vi "Drawer.vi"() -> ()   [LabVIEW 2014]
uses:
  <vilib>/Utility/file.llb/Read From Spreadsheet File (string).vi
  <vilib>/Utility/file.llb/Read From Spreadsheet File (I64).vi
  <vilib>/Utility/file.llb/Read From Spreadsheet File (DBL).vi
  <vilib>/Utility/file.llb/Write To Spreadsheet File (DBL).vi
  <vilib>/gmath/NI_Gmath.lvlib
panel:
  out "HF/LF slope":cluster{dbl[], dbl[]}[](graph)
  out "HF/LF flat":cluster{dbl[], dbl[]}[](graph)
  out "HF/LF_ERP 2":i32[][](graph)
  out "HF/LF_ERP":dbl[][](graph)
  out "HF_ERP":dbl[][](graph)
  out "LF_ERP":dbl[][](graph)
  out "VLF_ERP":dbl[][](graph)
  out "피험자_이름":string
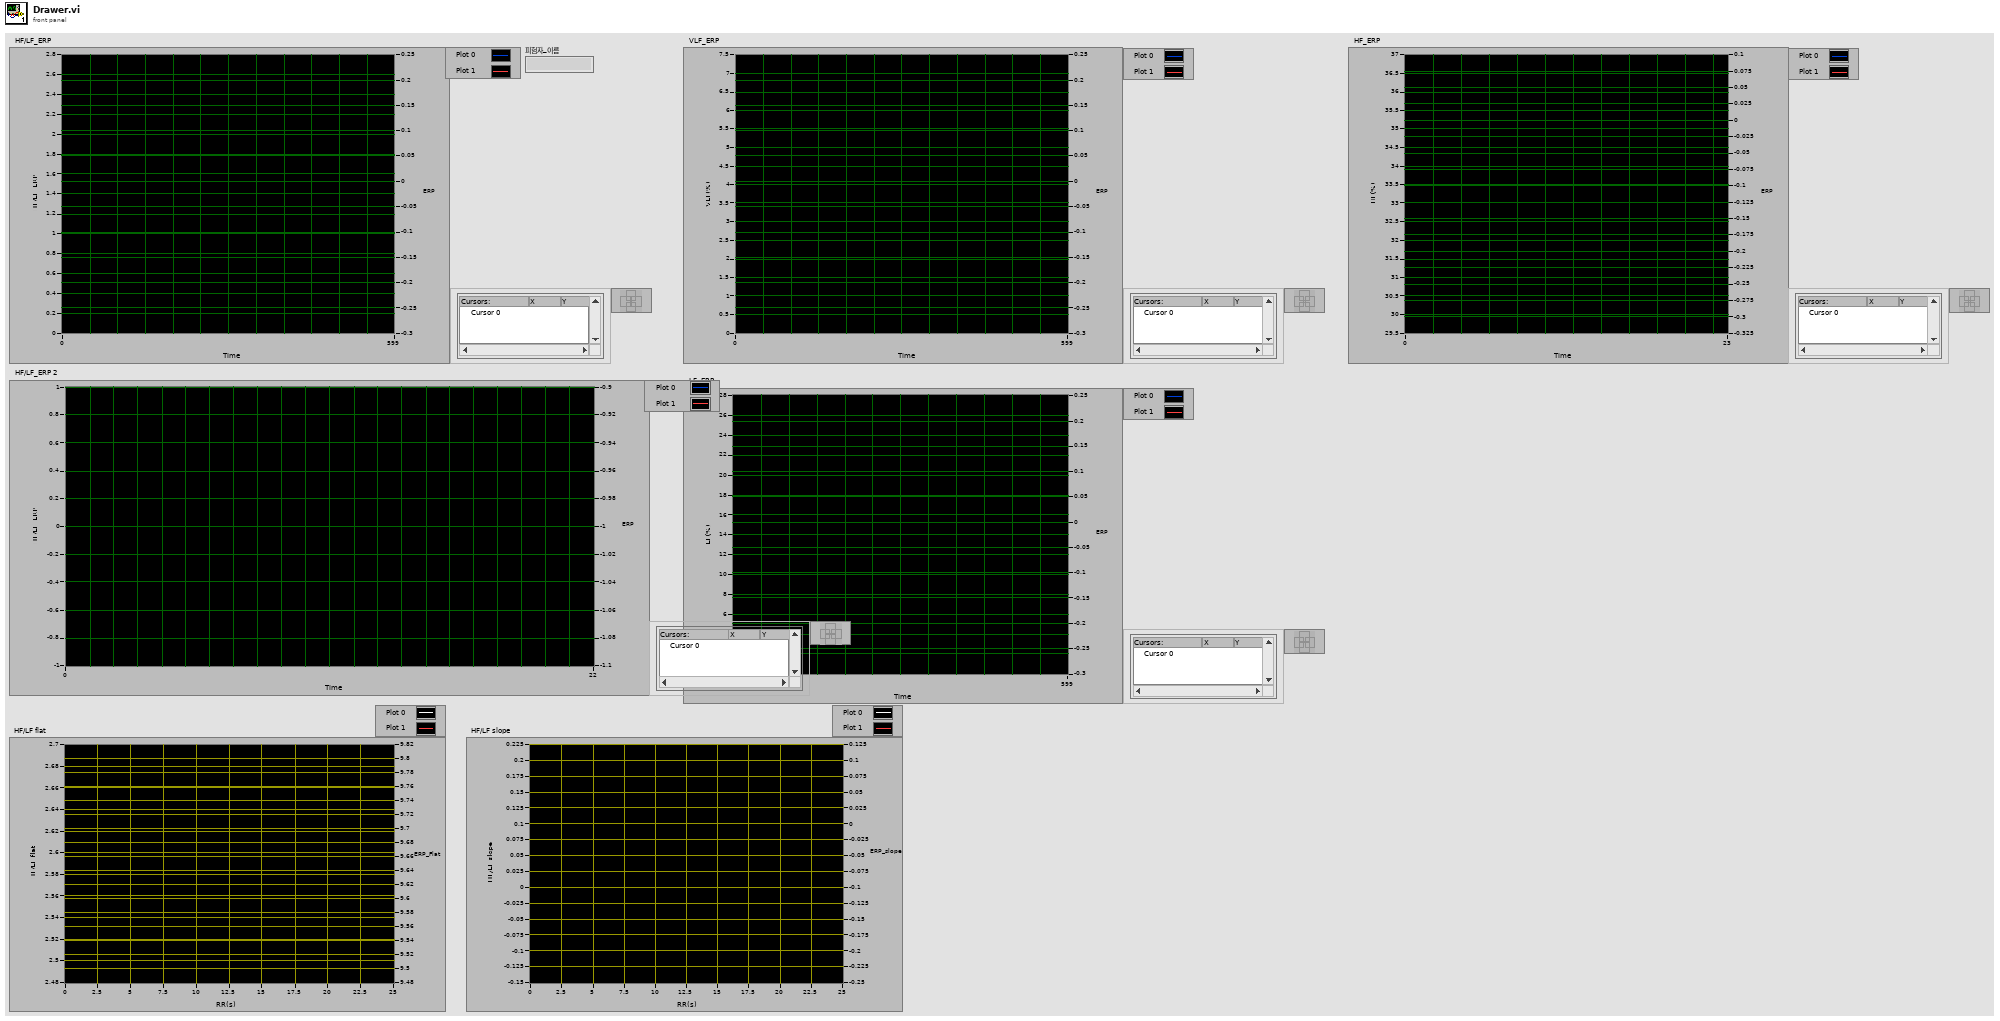
[diagram p1: front panel]
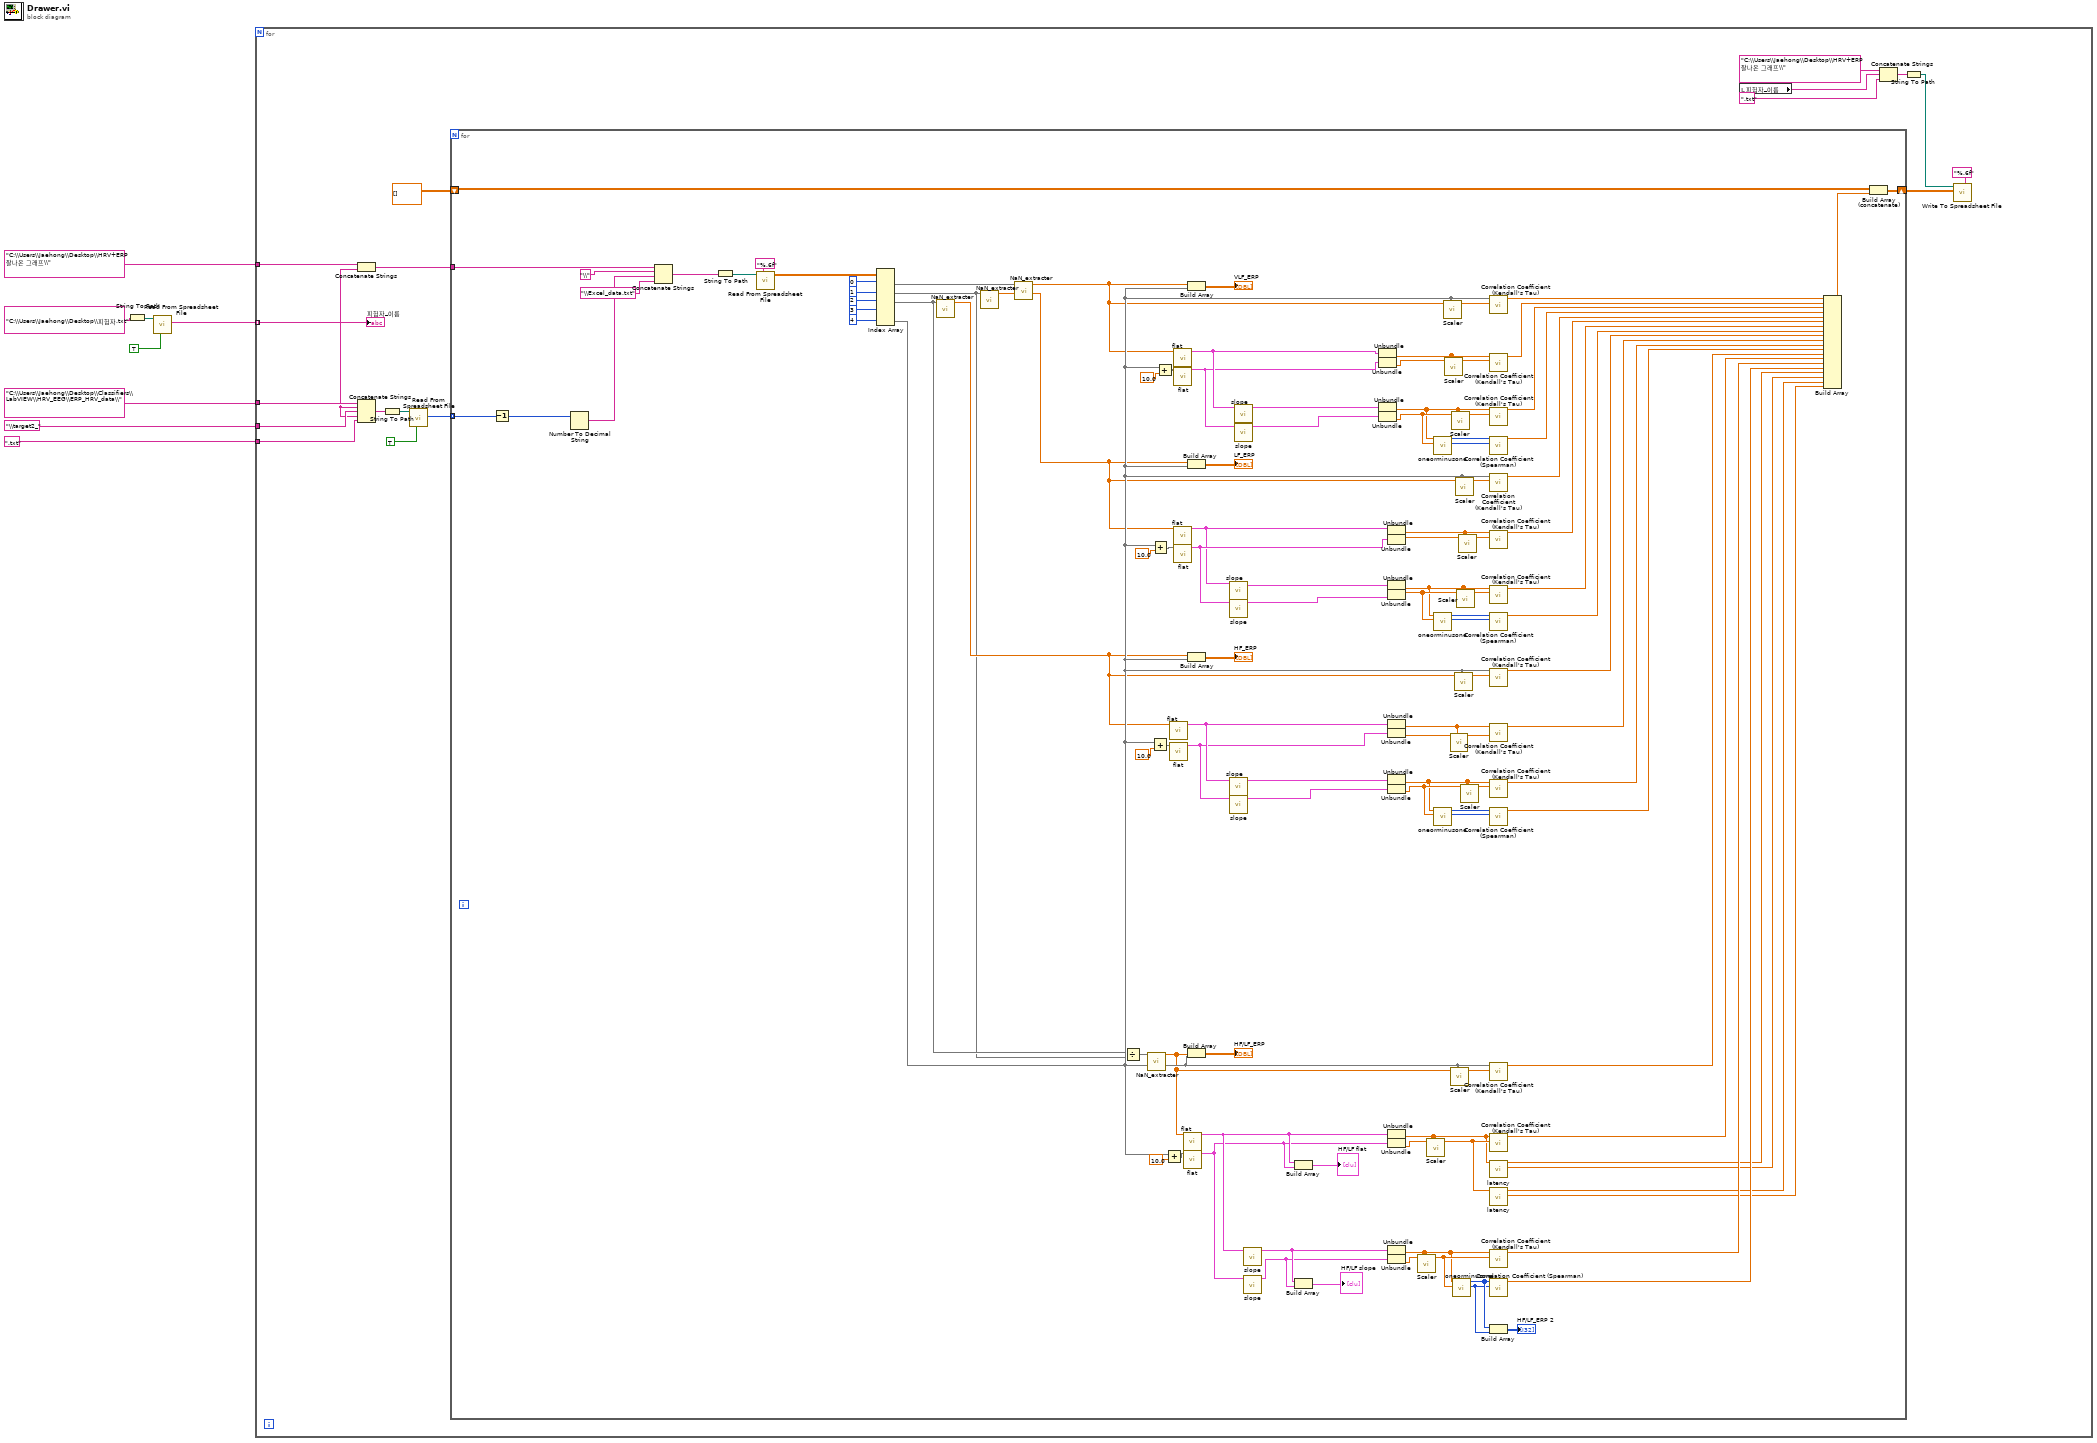
[diagram p0: block diagram]
diagram:
  n1 = String To Path(string="C:\\Users\\Jaehong\\Desktop\\피험자.txt") -> (path=w1:path)
  n2 = call-poly <vilib>:"Read From Spreadsheet File.vi"("transpose (no:F)"=TRUE, "file path (dialog if empty)"=w1) -> ("first row"=w3:string[])  [unwired: 5 in, 4 out]
  n3 = for {
    tunnel: "C:\\Users\\Jaehong\\Desktop\\HRV+ERP 잘나온 그래프\\" -> [w26]
    tunnel: "C:\\Users\\Jaehong\\Desktop\\Classifiers\\LabVIEW\\HRV_EEG\\ERP_HRV_data\\" -> [w24]
    tunnel: "\\target2_" -> [w23]
    tunnel: ".txt" -> [w22]
    tunnel: w3 -> [w18] mode=indexing
    n4 = Concatenate Strings(w26, w18) -> (w25:string)
    n5 = Concatenate Strings(w24, w18, w23, w18, w22) -> (w21:string)
    n6 = String To Path(string=w21) -> (path=w11:path)
    n7 = call-poly <vilib>:"Read From Spreadsheet File.vi"("transpose (no:F)"=TRUE, "file path (dialog if empty)"=w11) -> ("first row"=w9:i64[])  [unwired: 5 in, 4 out]
    n8 = for {
      tunnel: w25 -> [w140]
      shift-right: [w88] -> w19
      shift-left: dbl[][] [] -> [w103]
      tunnel: w9 -> [w42] mode=indexing
      n9 = Decrement(x=w42) -> (x-1=w41:i64)
      n10 = Number To Decimal String(number=w41) -> (decimal integer string=w138:string)  [unwired: 1 in]
      n11 = Concatenate Strings(w140, "\\", w138, "\\Excel_data.txt") -> (w136:string)
      n12 = String To Path(string=w136) -> (path=w135:path)
      n13 = call-poly <vilib>:"Read From Spreadsheet File.vi"("format (%.3f)"="%.6f", "file path (dialog if empty)"=w135) -> ("all rows"=w133:dbl[][])  [unwired: 5 in, 4 out]
      n14 = Index Array(array=w133, index (row) #1=0 ("index (row)"), index (row) #2=1 ("index (row)"), index (row) #3=2 ("index (row)"), index (row) #4=3 ("index (row)"), index (row) #5=4 ("index (row)")) -> (element #1=w43:dbl[], element #2=w29:dbl[], element #3=w31:dbl[], element #5=w46:dbl[])  [unwired: 5 in, 1 out]
      n15 = call "NaN_extracter.vi"("Array 1"=w31) -> ("Array 2"=w30:dbl[])  [unwired: 10 in]
      n16 = call "NaN_extracter.vi"("Array 1"=w29) -> ("Array 2"=w28:dbl[])  [unwired: 10 in]
      n17 = call "NaN_extracter.vi"("Array 1"=w43) -> ("Array 2"=w32:dbl[])  [unwired: 10 in]
      n18 = Divide(x=w31, y=w29) -> (x/y=w90:dbl[])
      n19 = call "NaN_extracter.vi"("Array 1"=w90) -> ("Array 2"=w27:dbl[])  [unwired: 10 in]
      n20 = Add(x=w46, y=10.0) -> (x+y=w121:dbl[])
      n21 = Add(x=w46, y=10.0) -> (x+y=w119:dbl[])
      n22 = Add(x=w46, y=10.0) -> (x+y=w117:dbl[])
      n23 = Add(x=w46, y=10.0) -> (x+y=w123:dbl[])
      n24 = call "flat.vi"("Input"=w30) -> ("XY Graph 3"=w107:cluster{dbl[], dbl[]})  [unwired: 10 in]
      n25 = call "flat.vi"("Input"=w121) -> ("XY Graph 3"=w106:cluster{dbl[], dbl[]})  [unwired: 10 in]
      n26 = call "flat.vi"("Input"=w32) -> ("XY Graph 3"=w115:cluster{dbl[], dbl[]})  [unwired: 10 in]
      n27 = call "flat.vi"("Input"=w117) -> ("XY Graph 3"=w114:cluster{dbl[], dbl[]})  [unwired: 10 in]
      n28 = call "flat.vi"("Input"=w28) -> ("XY Graph 3"=w110:cluster{dbl[], dbl[]})  [unwired: 10 in]
      n29 = call "flat.vi"("Input"=w119) -> ("XY Graph 3"=w111:cluster{dbl[], dbl[]})  [unwired: 10 in]
      n30 = call "flat.vi"("Input"=w27) -> ("XY Graph 3"=w71:cluster{dbl[], dbl[]})  [unwired: 10 in]
      n31 = call "flat.vi"("Input"=w123) -> ("XY Graph 3"=w70:cluster{dbl[], dbl[]})  [unwired: 10 in]
      n32 = Build Array(w32, w46) -> (→"VLF_ERP":dbl[][])
      n33 = Build Array(w28, w46) -> (→"LF_ERP":dbl[][])
      n34 = Build Array(w30, w46) -> (→"HF_ERP":dbl[][])
      n35 = Build Array(w27, w46) -> (→"HF/LF_ERP":dbl[][])
      n36 = call "slope.vi"("input"=w110) -> ("output"=w109:cluster{dbl[], dbl[]})  [unwired: 10 in]
      n37 = call "slope.vi"("input"=w111) -> ("output"=w108:cluster{dbl[], dbl[]})  [unwired: 10 in]
      n38 = call "slope.vi"("input"=w107) -> ("output"=w105:cluster{dbl[], dbl[]})  [unwired: 10 in]
      n39 = call "slope.vi"("input"=w106) -> ("output"=w104:cluster{dbl[], dbl[]})  [unwired: 10 in]
      n40 = call "slope.vi"("input"=w115) -> ("output"=w112:cluster{dbl[], dbl[]})  [unwired: 10 in]
      n41 = call "slope.vi"("input"=w114) -> ("output"=w113:cluster{dbl[], dbl[]})  [unwired: 10 in]
      n42 = call "slope.vi"("input"=w71) -> ("output"=w68:cluster{dbl[], dbl[]})  [unwired: 10 in]
      n43 = call "slope.vi"("input"=w70) -> ("output"=w67:cluster{dbl[], dbl[]})  [unwired: 10 in]
      n44 = Build Array(w71, w70) -> (→"HF/LF flat":cluster{dbl[], dbl[]}[])
      n45 = Build Array(w68, w67) -> (→"HF/LF slope":cluster{dbl[], dbl[]}[])
      n46 = Unbundle(w115) -> (w50:dbl[])  [unwired: 1 out]
      n47 = Unbundle(w114) -> (w102:dbl[])  [unwired: 1 out]
      n48 = Unbundle(w112) -> (w51:dbl[])  [unwired: 1 out]
      n49 = Unbundle(w113) -> (w101:dbl[])  [unwired: 1 out]
      n50 = Unbundle(w110) -> (w53:dbl[])  [unwired: 1 out]
      n51 = Unbundle(w111) -> (w98:dbl[])  [unwired: 1 out]
      n52 = Unbundle(w109) -> (w52:dbl[])  [unwired: 1 out]
      n53 = Unbundle(w108) -> (w97:dbl[])  [unwired: 1 out]
      n54 = Unbundle(w107) -> (w54:dbl[])  [unwired: 1 out]
      n55 = Unbundle(w106) -> (w94:dbl[])  [unwired: 1 out]
      n56 = Unbundle(w105) -> (w55:dbl[])  [unwired: 1 out]
      n57 = Unbundle(w104) -> (w93:dbl[])  [unwired: 1 out]
      n58 = Unbundle(w71) -> (w56:dbl[])  [unwired: 1 out]
      n59 = Unbundle(w70) -> (w65:dbl[])  [unwired: 1 out]
      n60 = Unbundle(w68) -> (w57:dbl[])  [unwired: 1 out]
      n61 = Unbundle(w67) -> (w86:dbl[])  [unwired: 1 out]
      n62 = call "Scaler.vi"("Array1"=w57, "Array2"=w86) -> ("Array_out"=w58:dbl[])  [unwired: 9 in]
      n63 = call "Scaler.vi"("Array1"=w56, "Array2"=w65) -> ("Array_out"=w59:dbl[])  [unwired: 9 in]
      n64 = call "oneorminusone.vi"("input 2"=w101, "input1"=w51) -> ("output2"=w99:i32[], "output1"=w100:i32[])  [unwired: 8 in]
      n65 = call "oneorminusone.vi"("input 2"=w97, "input1"=w52) -> ("output2"=w95:i32[], "output1"=w96:i32[])  [unwired: 8 in]
      n66 = call "oneorminusone.vi"("input 2"=w93, "input1"=w55) -> ("output2"=w91:i32[], "output1"=w92:i32[])  [unwired: 8 in]
      n67 = call "Scaler.vi"("Array1"=w46, "Array2"=w32) -> ("Array_out"=w49:dbl[])  [unwired: 9 in]
      n68 = call "Scaler.vi"("Array1"=w50, "Array2"=w102) -> ("Array_out"=w48:dbl[])  [unwired: 9 in]
      n69 = call "Scaler.vi"("Array1"=w54, "Array2"=w94) -> ("Array_out"=w62:dbl[])  [unwired: 9 in]
      n70 = call "Scaler.vi"("Array1"=w46, "Array2"=w27) -> ("Array_out"=w60:dbl[])  [unwired: 9 in]
      n71 = call "Scaler.vi"("Array1"=w51, "Array2"=w101) -> ("Array_out"=w47:dbl[])  [unwired: 9 in]
      n72 = call "oneorminusone.vi"("input 2"=w58, "input1"=w57) -> ("output2"=w72:i32[], "output1"=w73:i32[])  [unwired: 8 in]
      n73 = call "Scaler.vi"("Array1"=w46, "Array2"=w30) -> ("Array_out"=w63:dbl[])  [unwired: 9 in]
      n74 = call "Scaler.vi"("Array1"=w46, "Array2"=w28) -> ("Array_out"=w45:dbl[])  [unwired: 9 in]
      n75 = call "Scaler.vi"("Array1"=w52, "Array2"=w97) -> ("Array_out"=w64:dbl[])  [unwired: 9 in]
      n76 = call "Scaler.vi"("Array1"=w53, "Array2"=w98) -> ("Array_out"=w44:dbl[])  [unwired: 9 in]
      n77 = call "Scaler.vi"("Array1"=w55, "Array2"=w93) -> ("Array_out"=w61:dbl[])  [unwired: 9 in]
      n78 = call <vilib>:"Correlation Coefficient (Kendall's Tau).vi"("Y"=w49, "X"=w46) -> ("correlation coefficient r"=w89:dbl)  [unwired: 8 in, 1 out]
      n79 = call <vilib>:"Correlation Coefficient (Kendall's Tau).vi"("Y"=w48, "X"=w50) -> ("correlation coefficient r"=w85:dbl)  [unwired: 8 in, 1 out]
      n80 = call <vilib>:"Correlation Coefficient (Kendall's Tau).vi"("Y"=w47, "X"=w51) -> ("correlation coefficient r"=w84:dbl)  [unwired: 8 in, 1 out]
      n81 = call <vilib>:"Correlation Coefficient (Spearman).vi"("Y"=w99, "X"=w100) -> ("correlation coefficient r"=w83:dbl)  [unwired: 8 in, 1 out]
      n82 = call <vilib>:"Correlation Coefficient (Kendall's Tau).vi"("Y"=w45, "X"=w46) -> ("correlation coefficient r"=w82:dbl)  [unwired: 8 in, 1 out]
      n83 = call <vilib>:"Correlation Coefficient (Kendall's Tau).vi"("Y"=w44, "X"=w53) -> ("correlation coefficient r"=w81:dbl)  [unwired: 8 in, 1 out]
      n84 = call <vilib>:"Correlation Coefficient (Kendall's Tau).vi"("Y"=w64, "X"=w52) -> ("correlation coefficient r"=w80:dbl)  [unwired: 8 in, 1 out]
      n85 = call <vilib>:"Correlation Coefficient (Spearman).vi"("Y"=w95, "X"=w96) -> ("correlation coefficient r"=w79:dbl)  [unwired: 8 in, 1 out]
      n86 = call <vilib>:"Correlation Coefficient (Kendall's Tau).vi"("Y"=w63, "X"=w46) -> ("correlation coefficient r"=w78:dbl)  [unwired: 8 in, 1 out]
      n87 = call <vilib>:"Correlation Coefficient (Kendall's Tau).vi"("Y"=w62, "X"=w54) -> ("correlation coefficient r"=w77:dbl)  [unwired: 8 in, 1 out]
      n88 = call <vilib>:"Correlation Coefficient (Kendall's Tau).vi"("Y"=w61, "X"=w55) -> ("correlation coefficient r"=w76:dbl)  [unwired: 8 in, 1 out]
      n89 = call <vilib>:"Correlation Coefficient (Spearman).vi"("Y"=w91, "X"=w92) -> ("correlation coefficient r"=w75:dbl)  [unwired: 8 in, 1 out]
      n90 = call <vilib>:"Correlation Coefficient (Kendall's Tau).vi"("Y"=w60, "X"=w46) -> ("correlation coefficient r"=w40:dbl)  [unwired: 8 in, 1 out]
      n91 = call <vilib>:"Correlation Coefficient (Kendall's Tau).vi"("Y"=w59, "X"=w56) -> ("correlation coefficient r"=w39:dbl)  [unwired: 8 in, 1 out]
      n92 = call "latency.vi"("input"=w56) -> ("N1_latency"=w35:dbl, "P3_latency"=w36:dbl)  [unwired: 9 in]
      n93 = call "latency.vi"("input"=w59) -> ("N1_latency"=w33:dbl, "P3_latency"=w34:dbl)  [unwired: 9 in]
      n94 = call <vilib>:"Correlation Coefficient (Kendall's Tau).vi"("Y"=w58, "X"=w57) -> ("correlation coefficient r"=w38:dbl)  [unwired: 8 in, 1 out]
      n95 = call <vilib>:"Correlation Coefficient (Spearman).vi"("Y"=w72, "X"=w73) -> ("correlation coefficient r"=w37:dbl)  [unwired: 8 in, 1 out]
      n96 = Build Array(w73, w72) -> (→"HF/LF_ERP 2":i32[][])
      n97 = Build Array(w89, w85, w84, w83, w82, w81, w80, w79, w78, w77, w76, w75, w40, w39, w38, w37, w36, w35, w34, w33) -> (w87:dbl[])
      n98 = Build Array (concatenate)(w103, w87) -> (w88:dbl[][])
    }
    n99 = local read "피험자_이름"() -> (w16:string)
    n100 = Concatenate Strings("C:\\Users\\Jaehong\\Desktop\\HRV+ERP 잘나온 그래프\\", w16, ".txt") -> (w14:string)
    n101 = String To Path(string=w14) -> (path=w13:path)
    n102 = call-poly <vilib>:"Write To Spreadsheet File.vi"("format (%.3f)"="%.6f", "2D data"=w19, "file path (dialog if empty)"=w13) -> ()  [unwired: 5 in, 1 out]
    "피험자_이름" <- w18
  }
